vi "Configure Modulation Low Level (State).vi"(8 "error in (no error)":errorcluster, 9 "Enable (F: Off)":bool, 10 "Modulation (AM)":enum16{"AM", "FM", "PM", "FSK", "PWM"}(ring), 11 "VISA resource name":refnum<visa-resource-name>) -> (0 "error out":errorcluster, 3 "VISA resource name out":refnum<visa-resource-name>)   [LabVIEW 2017, in "Keithley 3390.lvlib"]
uses:
  Keithley 3390.lvlib
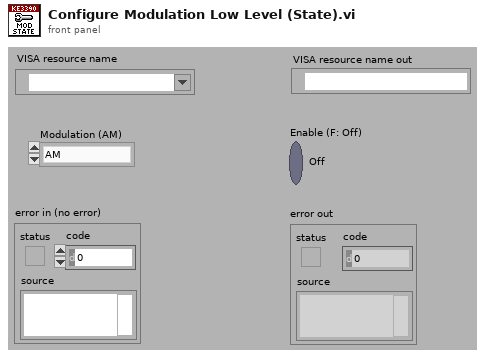
[diagram p1: front panel]
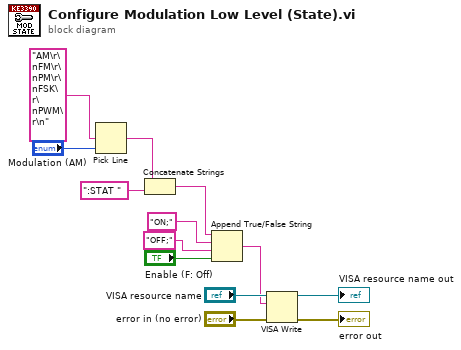
[diagram p0: block diagram]
diagram:
  n1 = Pick Line(multi-line string="AM\r\nFM\r\nPM\r\nFSK\r\nPWM\r\n" ("options"), line index="Modulation (AM)") -> (output string=w10:string)  [unwired: 1 in]
  n2 = Concatenate Strings(w10, ":STAT " ("command")) -> (w4:string)
  n3 = Append True/False String(1:"Enable (F: Off)", 2:"OFF;" ("false string"), 3:"ON;" ("true string"), 4:w4) -> (0:w5:string)
  n4 = VISA Write(VISA resource name="VISA resource name", write buffer=w5, error in (no error)="error in (no error)") -> (VISA resource name out=→"VISA resource name out":refnum<visa-resource-name>, error out=→"error out":errorcluster)  [unwired: 1 out]
